vi "Payload to Long.vi"(3 "Payload":string) -> (1 "Long":i32[](array[numeric]))   [LabVIEW 2019]
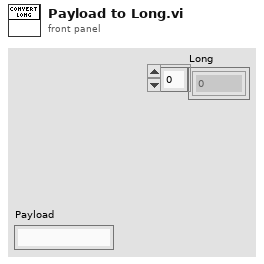
[diagram p1: front panel]
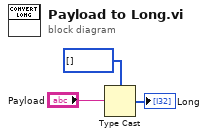
[diagram p0: block diagram]
diagram:
  n1 = Type Cast(type=i32[] [] ("Data"), x="Payload") -> (*(type *) &x=→"Long":i32[])
